vi "FlatToRichcif_manager_LauncherStatus.vi"(5 "OutputClusterType":T1, 11 "InputCluster":T5) -> (3 "OutputCluster":T1)   [LabVIEW 2021, in "CIF_Manager_client.lvlib"]
uses:
  CIF_Manager_client.lvlib
  cif_manager_LauncherStatus_Flat.ctl
  cif_manager_LauncherInfo_Flat.ctl
  cif_manager_LauncherType.ctl
  cif_common_Status_Flat.ctl
  cif_manager_LauncherStatus.ctl
  cif_manager_LauncherInfo.ctl
  cif_common_Status.ctl
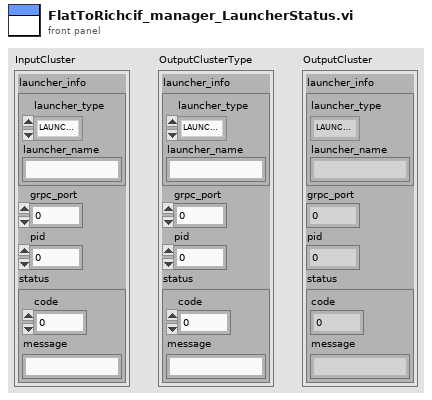
[diagram p1: front panel]
types:
  T1 = typedef "CIF_Manager_client.lvlib/cif_manager_LauncherStatus.ctl" = cluster{"launcher_info":T2, "grpc_port":i32, "pid":u32, "status":T4}
  T2 = typedef "CIF_Manager_client.lvlib/cif_manager_LauncherInfo.ctl" = cluster{"launcher_type":T3, "launcher_name":string}
  T3 = typedef "CIF_Manager_client.lvlib/cif_manager_LauncherType.ctl" = enum32{"LAUNCHERTYPE_UNKNOWN", "LAUNCHERTYPE_LABVIEW"}
  T4 = typedef "CIF_Manager_client.lvlib/cif_common_Status.ctl" = cluster{"code":i32, "message":string}
  T5 = typedef "CIF_Manager_client.lvlib/cif_manager_LauncherStatus_Flat.ctl" = cluster{"launcher_info":T6, "grpc_port":i32, "pid":u32, "status":T7}
  T6 = typedef "CIF_Manager_client.lvlib/cif_manager_LauncherInfo_Flat.ctl" = cluster{"launcher_type":T3, "launcher_name":string}
  T7 = typedef "CIF_Manager_client.lvlib/cif_common_Status_Flat.ctl" = cluster{"code":i32, "message":string}
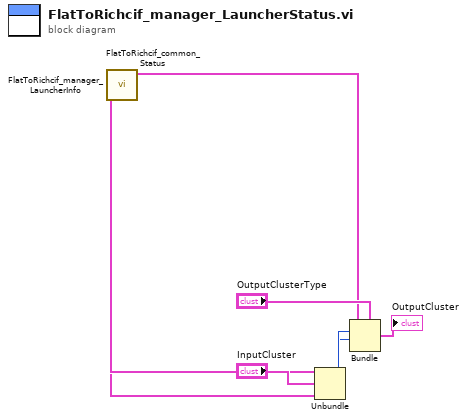
[diagram p0: block diagram]
diagram:
  n1 = Unbundle "Unbundle"("InputCluster") -> ("launcher_info"=w6:T6, "grpc_port"=w4:i32, "pid"=w3:u32, "status"=w2:T7)
  n2 = call "FlatToRichcif_common_Status.vi"("InputCluster"=w2) -> ("OutputCluster"=w1:T4)  [unwired: 10 in]
  n3 = call "FlatToRichcif_manager_LauncherInfo.vi"("InputCluster"=w6) -> ("OutputCluster"=w5:T2)  [unwired: 10 in]
  n4 = Bundle "Bundle"(cluster="OutputClusterType", "launcher_info"=w5, "grpc_port"=w4, "pid"=w3, "status"=w1) -> (→"OutputCluster":T1)
